vi "Logger Initialize.vi"(0 "Queue Name":string="Station Status", 5 "Server Status":enum16{"Running", "Closed"}(ring), 11 "error in (no error)":errorcluster) -> (15 "error out":errorcluster)   [LabVIEW 2018]
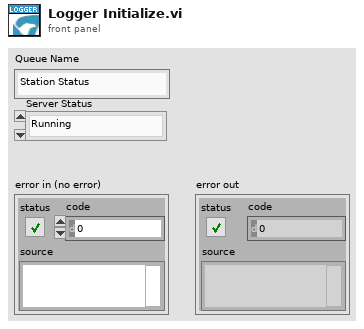
[diagram p1: front panel]
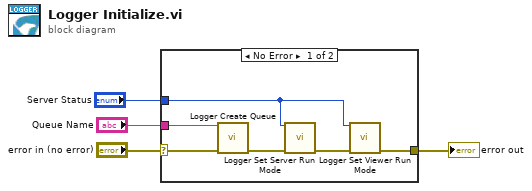
[diagram p0: block diagram]
diagram:
  n1 = case shown="No Error" "error in (no error)" {
    selector: "error in (no error)" -> [w10 w11]
    tunnel: [w6 w11] -> w3
    tunnel: "Queue Name" -> [w9 _]
    tunnel: "Server Status" -> [w5 _]
    frame No Error {
      n2 = call "Logger Create Queue.vi"("Queue Name"=w9, "error in (no error)"=w10) -> ("error out"=w8:errorcluster)  [unwired: 12 in, 1 out]
      n3 = call "Logger Set Server Run Mode.vi"("Server Status"=w5, "error in (no error)"=w8) -> ("error out"=w7:errorcluster)  [unwired: 13 in]
      n4 = call "Logger Set Viewer Run Mode.vi"("Server Status"=w5, "error in (no error)"=w7) -> ("error out"=w6:errorcluster)  [unwired: 13 in]
    }
    frame Error {
    }
  }
  "error out" <- w3
